vi "Create Panel.vi"(10 "Actor":refnum<class "Actor.lvclass">, 11 "Panel in":refnum<class "Panel.lvclass">) -> (0 "error out":errorcluster, 3 "Panel out":refnum<class "Panel.lvclass">)   [LabVIEW 2021, in "Panel.lvclass"]
uses:
  Panel.lvclass
  LVCAM/LVCAM/Actor/Actor.lvclass
  Panel Wrapper.vi
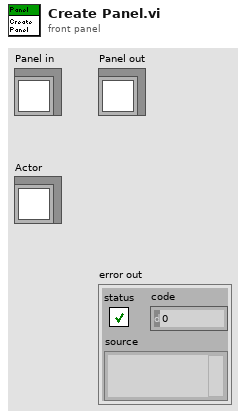
[diagram p1: front panel]
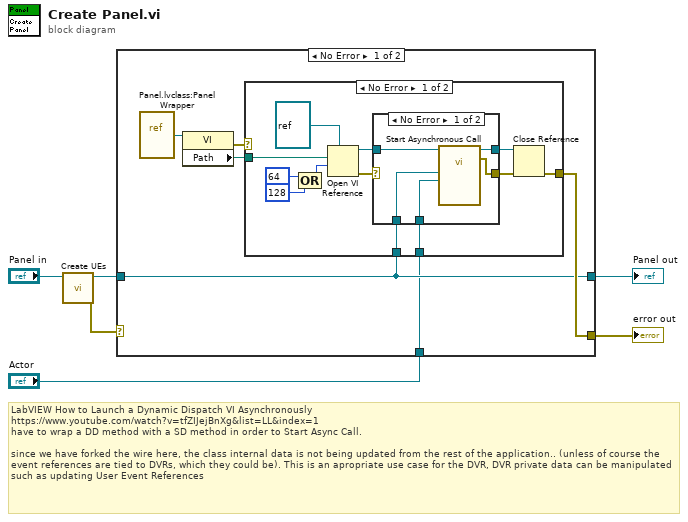
[diagram p0: block diagram]
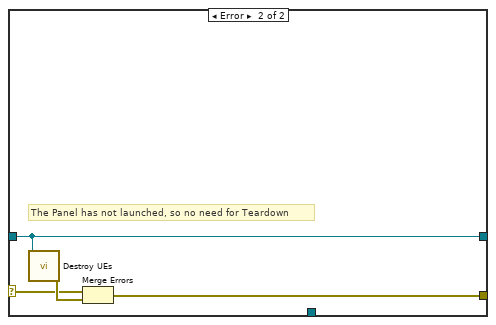
[diagram p4: hidden frame]
diagram:
  # "LabVIEW How to Launch a Dynamic Dispatch VI Asynchronously\nhttps://www.youtube.com/watch?v=tfZIJejBnXg&list=LL&index=1\nhave to wrap a DD method with a SD method in order to Start Async Call.\n\nsince we have forked the wire here, the class internal data is not being updated from the rest of the application.. (unless of course the event references are tied to DVRs, which they could be). This is an apropriate use case for the DVR, DVR private data can be manipulated such as updating User Event References"
  n1 = call-dynamic "Create UEs.vi"("Panel in"="Panel in") -> ("error out"=w6:errorcluster, "Panel out"=w5:refnum<class "Panel.lvclass">)  [unwired: 9 in]
  n2 = case shown="No Error" w6 {
    selector: w6 -> [_ w33]
    tunnel: [w9 w36] -> w1
    tunnel: w5 -> [w8 w34]
    tunnel: [w8 w34] -> w2
    tunnel: "Actor" -> [w7 _]
    frame No Error {
      n3 = vi-ref "Panel.lvclass:Panel Wrapper.vi"() -> (w11:refnum<vi>)
      n4 = property class="VI"(reference=w11) -> (error out=w12:errorcluster, "Path"=w10:path)  [unwired: 1 in, 1 out]
      n5 = case shown="No Error" w12 {
        selector: w12 -> [_ w32]
        tunnel: [w22 w32] -> w9
        tunnel: w10 -> [w18 _]
        tunnel: w8 -> [w14 _]
        tunnel: w7 -> [w13 _]
        frame No Error {
          n6 = Compound Arithmetic op=OR(64 ("options: Multiple Clones,\n  Fire & Forget"), 128 ("options: Multiple Clones,\n  Fire & Forget")) -> (w20:i32)
          n7 = Open VI Reference(type specifier VI Refnum (for type only)=refnum<vi> refnum, vi path=w18, options=w20) -> (vi reference=w16:refnum<vi>, error out=w17:errorcluster)  [unwired: 3 in]
          n8 = case shown="No Error" w17 {
            selector: w17 -> [_ w31]
            tunnel: [w29 w30] -> w24
            tunnel: [w28 w31] -> w23
            tunnel: w16 -> [w27 w30]
            tunnel: w14 -> [w26 _]
            tunnel: w13 -> [w25 _]
            frame No Error {
              n9 = call-by-ref "Start Asynchronous Call"(reference=w27, "LVCAM"=w25, "Panel in"=w26) -> (reference out=w29:refnum<vi>, error out=w28:errorcluster)  [unwired: 11 in]
            }
            frame Error {
            }
          }
          n10 = Close Reference(reference=w24, error in (no error)=w23) -> (error out=w22:errorcluster)
        }
        frame Error {
        }
      }
    }
    frame Error {
      # "The Panel has not launched, so no need for Teardown"
      n11 = call-dynamic "Destroy UEs.vi"("Panel in"=w34) -> ("error out"=w35:errorcluster)  [unwired: 10 in]
      n12 = Merge Errors(w33, w35) -> (w36:errorcluster)
    }
  }
  "error out" <- w1
  "Panel out" <- w2
